vi "Scaffold Saveas.vi"(11 "Item Ref":T1) -> ()   [LabVIEW 2012, in "Negentropic IDE.lvlib"]
uses:
  Negentropic IDE.lvlib
  <resource>/Framework/Providers/API/ItemRef.ctl
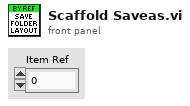
[diagram p1: front panel]
types:
  T1 = typedef "ItemRef.ctl" = u64
  T2 = typedef "Negentropic IDE.lvlib/Folder Config.ctl" = cluster{"Path":string, "Scope":T3}
  T3 = typedef "Negentropic IDE.lvlib/Scope.ctl" = enum32{"invalid scope", "public", "private", "protected", "community"}
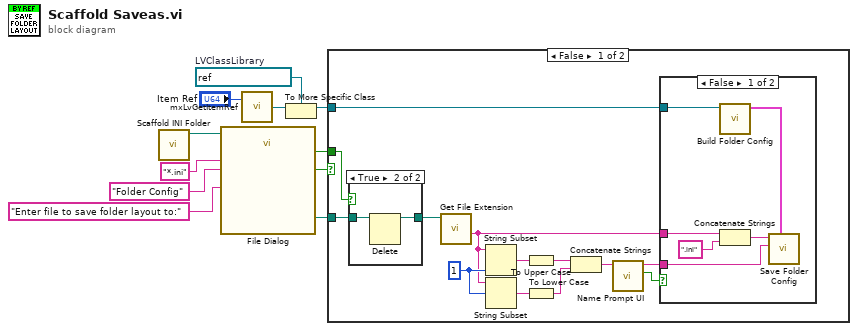
[diagram p0: block diagram]
diagram:
  w9 = refnum<vi> refnum  # LVClassLibrary
  n1 = call "Scaffold INI Folder.vi"() -> ("Scaffold INI Folder"=w8:path)  [unwired: 10 in, 1 out]
  n2 = call "File Dialog"("start path"=w8, "prompt"="Enter file to save folder layout to:", "pattern (all files)"="*.ini", "pattern label"="Folder Config" ("pattern (all files)")) -> ("selected path"=w4:path, "exists"=w2:bool, "cancelled"=w3:bool)  [unwired: 8 in, 1 out]
  n3 = call <resource>:"mxLvGetItemRef.vi"("Item"="Item Ref") -> ("Item Refnum"=w10:refnum<vi>)  [unwired: 1 in, 2 out]
  n4 = To More Specific Class(target class=w9, reference=w10) -> (specific class reference=w1:refnum<vi>)  [unwired: 1 in, 1 out]
  n5 = case shown="False" w3 {
    tunnel: w4 -> [w23 _]
    tunnel: w2 -> [w24 _]
    tunnel: w1 -> [w12 _]
    frame False {
      w20 = 1 ("length (rest)")
      n6 = case shown="True" w24 {
        tunnel: w23 -> [w31 w33]
        tunnel: [w31 w32] -> w22
        frame False {
        }
        frame True {
          n7 = Delete(path (use dialog)=w33) -> (deleted path=w32:path)  [unwired: 4 in, 2 out]
        }
      }
      n8 = call <vilib>:"Get File Extension.vi"("file"=w22) -> ("filename without extension"=w13:string)  [unwired: 6 in, 4 out]
      n9 = String Subset(string=w13, length (rest)=w20) -> (substring=w21:string)  [unwired: 1 in]
      n10 = String Subset(string=w13, offset (0)=w20) -> (substring=w19:string)  [unwired: 1 in]
      n11 = To Upper Case(1:w21) -> (0:w18:string)
      n12 = To Lower Case(string=w19) -> (all lower case string=w17:string)
      n13 = Concatenate Strings(w18, w17) -> (w16:string)
      n14 = call "Name Prompt UI.vi"("Initial Name (Empty)"=w16) -> ("Cancelled"=w15:bool, "Name"=w14:string)  [unwired: 9 in]
      n15 = case shown="False" w15 {
        tunnel: w14 -> [w27 _]
        tunnel: w13 -> [w30 _]
        tunnel: w12 -> [w26 _]
        frame False {
          n16 = call "Build Folder Config.vi"("Library"=w26) -> ("Folders"=w25:T2[])  [unwired: 10 in]
          n17 = Concatenate Strings(w30, ".ini" ("string")) -> (w28:string)
          n18 = call "Save Folder Config.vi"("Folder Config"=w25, "Name"=w27, "INI Filename"=w28) -> ()  [unwired: 8 in, 1 out]
        }
        frame True {
        }
      }
    }
    frame True {
    }
  }
